vi "__init__.vi"(8 "error in (no error)":errorcluster, 11 "self in":refnum<class "BlockId.lvclass">) -> (0 "error out":errorcluster, 3 "self out":refnum<class "BlockId.lvclass">)   [LabVIEW 2020, in "mlir.lvlib" / "BlockId.lvclass"]
uses:
  BlockId.lvclass
  BlockId.lvclass/BlockId.ctl
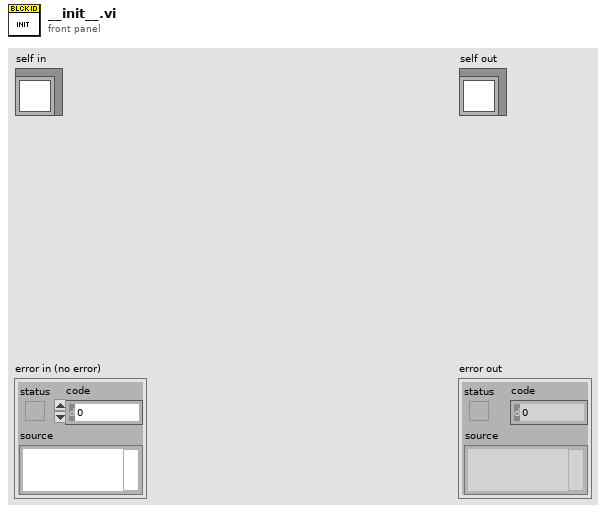
[diagram p1: front panel]
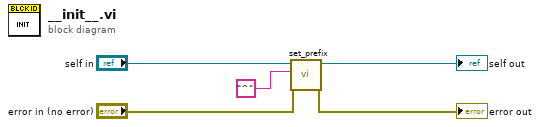
[diagram p0: block diagram]
diagram:
  n1 = call-dynamic "set_prefix.vi"("error in (no error)"="error in (no error)", "_prefix_"="^", "Identifier in"="self in") -> ("error out"=→"error out":errorcluster, "Identifier out"=→"self out":refnum<class "BlockId.lvclass">)  [unwired: 7 in]
